vi "map_roi.vi"(8 "Error In":errorcluster, 9 "Image Properties":T2, 10 "Parameters":T1, 11 "ROI In":T3) -> (0 "Error Out":errorcluster, 3 "ROI Out":T3)   [LabVIEW 2019]
uses:
  image_property_cluster_typedef.ctl
  parameters_cluster_typedef.ctl
  xi_angles_enum_typedef.ctl
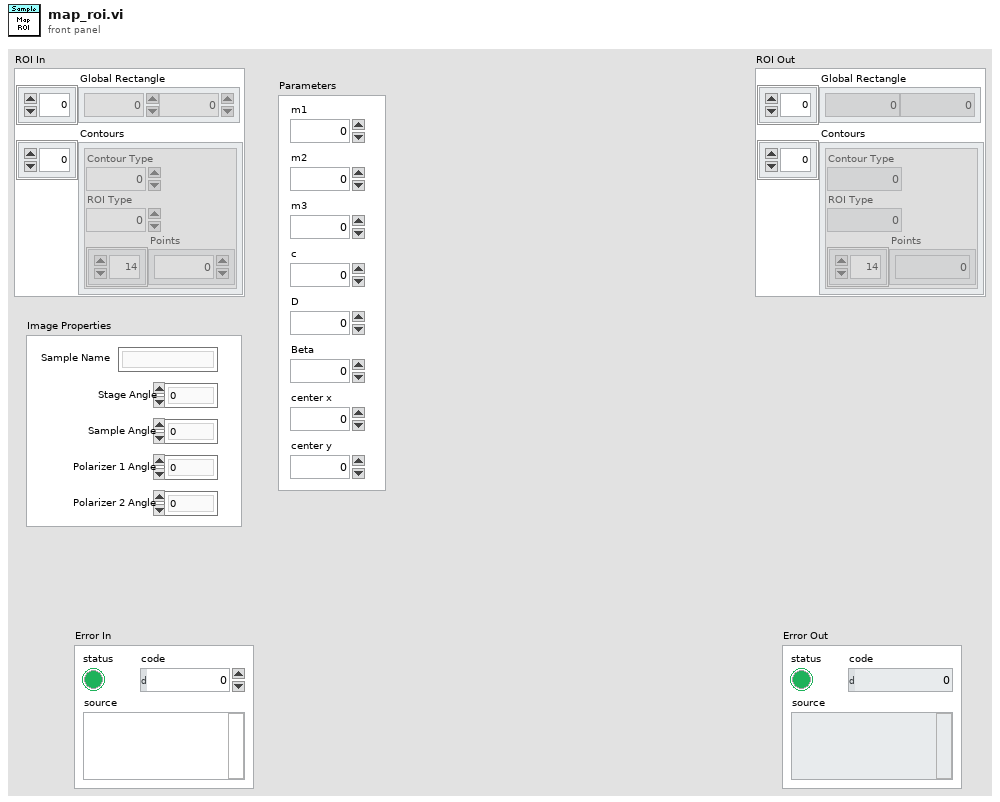
[diagram p1: front panel]
types:
  T1 = typedef "parameters_cluster_typedef.ctl" = cluster{"m1":dbl, "m2":dbl, "m3":dbl, "c":dbl, "D":dbl, "Beta":dbl, "center x":dbl, "center y":dbl}
  T2 = typedef "image_property_cluster_typedef.ctl" = cluster{"Stage Angle":dbl, "Sample Angle":dbl, "Polarizer 1 Angle":dbl, "Polarizer 2 Angle":dbl, "Sample Name":string}
  T3 = cluster{"Global Rectangle":i32[], "Contours":cluster{"Contour Type":u32, "ROI Type":u32, "Points":i32[]}[]}
  T4 = cluster{"Contour Type":u32, "ROI Type":u32, "Points":i32[]}
  T5 = typedef "xi_angles_enum_typedef.ctl" = enum16{"0", "45"}
  T6 = cluster{"Contour Type":u32, "ROI Type":u32, "Points":i32[]}[]
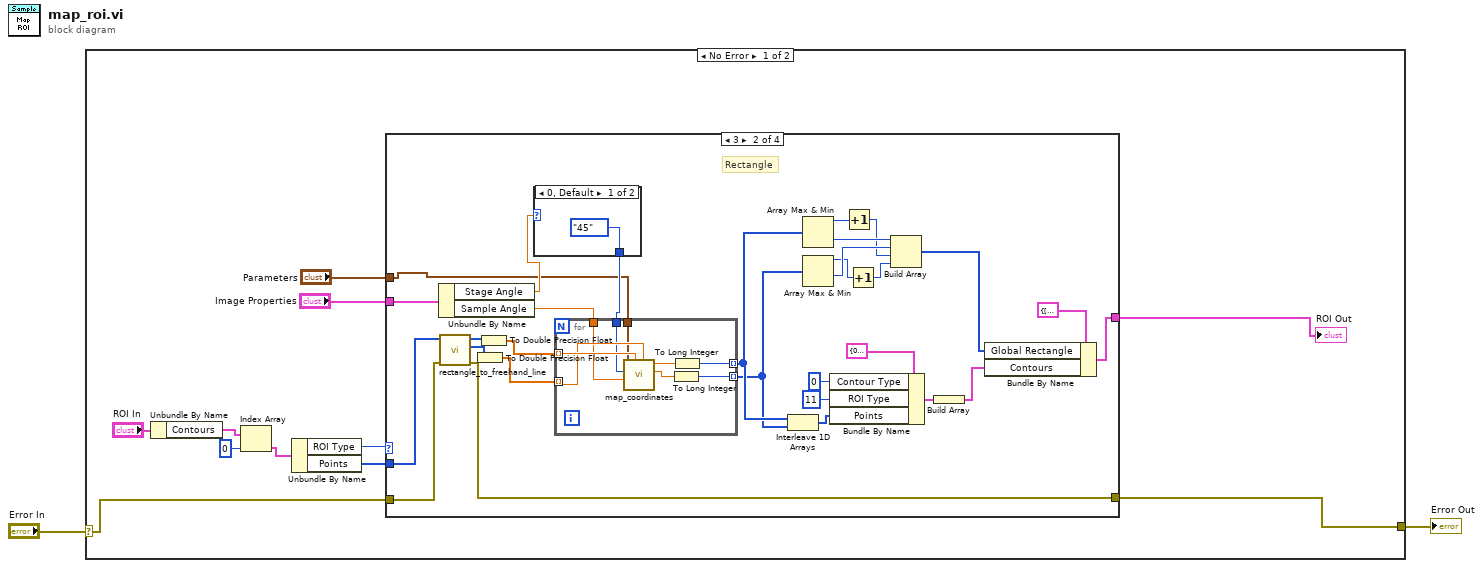
[diagram p0: block diagram]
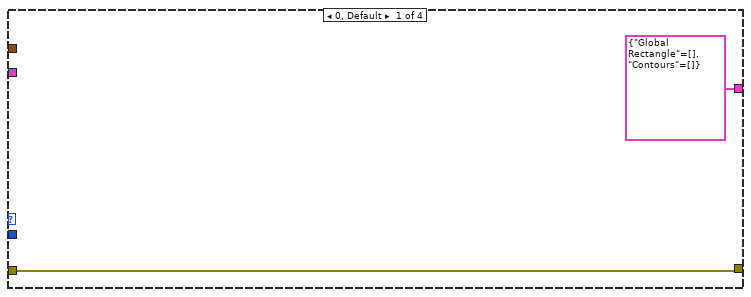
[diagram p2: hidden frame]
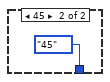
[diagram p3: hidden frame]
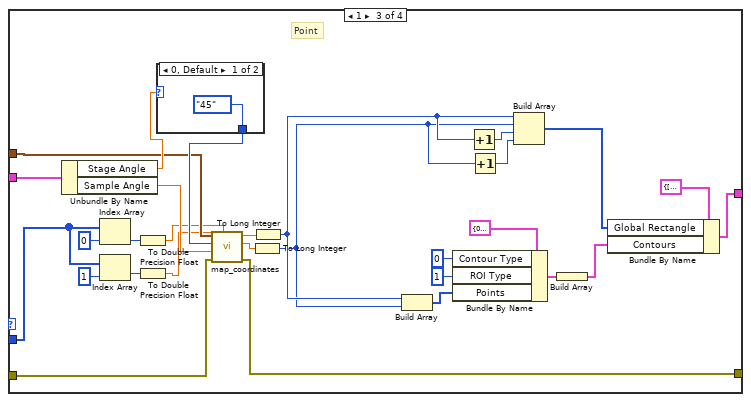
[diagram p4: hidden frame]
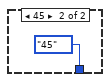
[diagram p5: hidden frame]
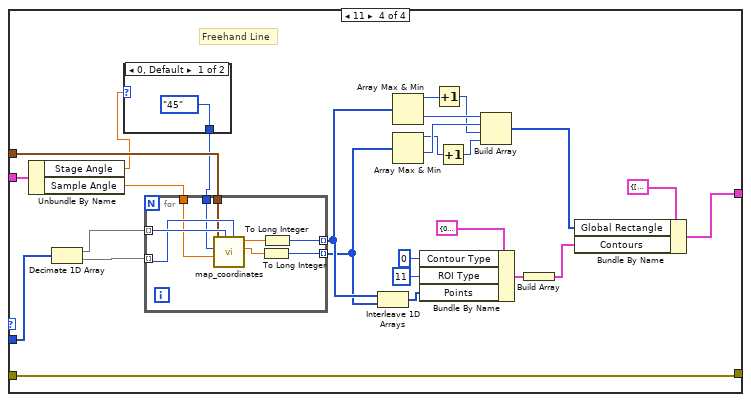
[diagram p6: hidden frame]
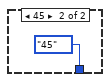
[diagram p7: hidden frame]
diagram:
  n1 = case shown="No Error" "Error In" {
    selector: "Error In" -> [w4 w124]
    tunnel: [w3 w124] -> w1
    frame No Error {
      n2 = Unbundle By Name("ROI In") -> ("Contours"=w12:T6)
      n3 = Index Array(array=w12, index=0) -> (element=w10:T4)
      n4 = Unbundle By Name(w10) -> ("ROI Type"=w9:u32, "Points"=w8:i32[])
      n5 = case shown="3" w9 {
        tunnel: w8 -> [_ w44 w72 w112]
        tunnel: "Parameters" -> [_ w23 w73 w107]
        tunnel: "Image Properties" -> [_ w22 w76 w109]
        tunnel: [T3 {"Global Rectangle"=[], "Contours"=[]} ("ROI Out") w17 w57 w105] -> w5
        tunnel: w4 -> [w14 w43 w65 w87]
        tunnel: [w14 w16 w56 w87] -> w3
        frame 0, Default {
        }
        frame 3 {
          # "Rectangle"
          n6 = Unbundle By Name(w22) -> ("Stage Angle"=w25:dbl, "Sample Angle"=w42:dbl)
          n7 = call "rectangle_to_freehand_line.vi"("Error In"=w43, "Input Rect"=w44) -> ("Error Out"=w16:errorcluster, "y"=w20:i32[], "x"=w21:i32[])  [unwired: 7 in]
          n8 = To Double Precision Float(number=w20) -> (double precision float=w18:dbl[])
          n9 = To Double Precision Float(number=w21) -> (double precision float=w19:dbl[])
          n10 = case shown="0, Default" w25 {
            tunnel: [xi_angles_enum_typedef."45" ("Xi From") xi_angles_enum_typedef."45" ("Xi From")] -> w24
            frame 0, Default {
            }
            frame 45 {
            }
          }
          n11 = for {
            tunnel: w19 -> [w55] mode=indexing
            tunnel: w18 -> [w54] mode=indexing
            tunnel: w42 -> [w53]
            tunnel: [w50] -> w34 mode=indexing
            tunnel: [w49] -> w33 mode=indexing
            tunnel: w23 -> [w48]
            tunnel: w24 -> [w47]
            n12 = call "map_coordinates.vi"("b"=w54, "a"=w55, "phi_in"=w53, "Xi From"=w47, "Parameters"=w48) -> ("b_pixel"=w51:dbl, "a_pixel"=w52:dbl)  [unwired: 4 in, 1 out]
            n13 = To Long Integer(number=w51) -> (32bit integer=w49:i32)
            n14 = To Long Integer(number=w52) -> (32bit integer=w50:i32)
          }
          n15 = Interleave 1D Arrays(w34, w33) -> (w37:i32[])
          n16 = Array Max & Min(array=w34) -> (max value=w30:i32, min value=w32:i32)  [unwired: 2 out]
          n17 = Array Max & Min(array=w33) -> (max value=w28:i32, min value=w31:i32)  [unwired: 2 out]
          n18 = Bundle By Name(cluster=T4 {"Contour Type"=0, "ROI Type"=0, "Points"=[]} ("Cluster"), "Contour Type"=u32 0, "ROI Type"=u32 11, "Points"=w37) -> (w36:T4)
          n19 = Increment(x=w30) -> (x+1=w29:i32)
          n20 = Increment(x=w28) -> (x+1=w27:i32)
          n21 = Build Array(w32, w31, w29, w27) -> (w26:i32[])
          n22 = Build Array(w36) -> (w35:T6)
          n23 = Bundle By Name(cluster=T3 {"Global Rectangle"=[387, 507, 423, 523], "Contours"=[{"Contour Type"=0, "ROI Type"=11, "Points"=[387, 521, 387, 520, 387, 519, 387, 518, 387, 517, 387, 516, 388, 516, 388, 515, 388, 514, 388, 513, 388, 512, 389, 512, 389, 511, 390, 511, 390, 510, 391, 510, 392, 510, 392, 509, 393, 509, 393, 508, 394, 508, 395, 508, 395, 507, 396, 507, 397, 507, 398, 508, 399, 508, 399, 509, 400, 509, 401, 509, 402, 509, 403, 509, 404, 509, 404, 510, 405, 510, 406, 510, 407, 510, 408, 510, 409, 510, 410, 510, 411, 510, 412, 510, 413, 510, 413, 511, 414, 511, 415, 511, 416, 511, 417, 512, 418, 512, 419, 512, 419, 513, 419, 514, 420, 514, 421, 514, 421, 515, 421, 516, 422, 517, 422, 518, 422, 519, 421, 519, 421, 520, 420, 520, 419, 520, 418, 520, 417, 520, 416, 520, 415, 520, 414, 520, 413, 520, 412, 520, 411, 520, 410, 520, 409, 520, 409, 521, 408, 521, 407, 521, 406, 521, 405, 521, 404, 521, 403, 521, 402, 521, 401, 521, 400, 521, 399, 521, 398, 521, 398, 522, 397, 522, 396, 522, 395, 522, 394, 522, 393, 522, 392, 522, 391, 522, 390, 522, 389, 522, 389, 522]}]} ("ROI Out"), "Global Rectangle"=w26, "Contours"=w35) -> (w17:T3)
        }
        frame 1 {
          # "Point"
          n24 = Unbundle By Name(w76) -> ("Stage Angle"=w77:dbl, "Sample Angle"=w75:dbl)
          n25 = Index Array(array=w72, index=0) -> (element=w69:i32)
          n26 = Index Array(array=w72, index=1) -> (element=w68:i32)
          n27 = To Double Precision Float(number=w69) -> (double precision float=w67:dbl)
          n28 = To Double Precision Float(number=w68) -> (double precision float=w66:dbl)
          n29 = case shown="0, Default" w77 {
            tunnel: [xi_angles_enum_typedef."45" ("Xi From") xi_angles_enum_typedef."45" ("Xi From")] -> w74
            frame 0, Default {
            }
            frame 45 {
            }
          }
          n30 = call "map_coordinates.vi"("b"=w66, "a"=w67, "Error In"=w65, "phi_in"=w75, "Xi From"=w74, "Parameters"=w73) -> ("Error Out"=w56:errorcluster, "b_pixel"=w63:dbl, "a_pixel"=w64:dbl)  [unwired: 3 in]
          n31 = To Long Integer(number=w63) -> (32bit integer=w58:i32)
          n32 = To Long Integer(number=w64) -> (32bit integer=w59:i32)
          n33 = Build Array(w59, w58) -> (w60:i32[])
          n34 = Bundle By Name(cluster=T4 {"Contour Type"=0, "ROI Type"=0, "Points"=[]} ("Cluster"), "Contour Type"=u32 0, "ROI Type"=u32 1, "Points"=w60) -> (w80:T4)
          n35 = Increment(x=w59) -> (x+1=w61:i32)
          n36 = Increment(x=w58) -> (x+1=w62:i32)
          n37 = Build Array(w59, w58, w61, w62) -> (w78:i32[])
          n38 = Build Array(w80) -> (w79:T6)
          n39 = Bundle By Name(cluster=T3 {"Global Rectangle"=[387, 507, 423, 523], "Contours"=[{"Contour Type"=0, "ROI Type"=11, "Points"=[387, 521, 387, 520, 387, 519, 387, 518, 387, 517, 387, 516, 388, 516, 388, 515, 388, 514, 388, 513, 388, 512, 389, 512, 389, 511, 390, 511, 390, 510, 391, 510, 392, 510, 392, 509, 393, 509, 393, 508, 394, 508, 395, 508, 395, 507, 396, 507, 397, 507, 398, 508, 399, 508, 399, 509, 400, 509, 401, 509, 402, 509, 403, 509, 404, 509, 404, 510, 405, 510, 406, 510, 407, 510, 408, 510, 409, 510, 410, 510, 411, 510, 412, 510, 413, 510, 413, 511, 414, 511, 415, 511, 416, 511, 417, 512, 418, 512, 419, 512, 419, 513, 419, 514, 420, 514, 421, 514, 421, 515, 421, 516, 422, 517, 422, 518, 422, 519, 421, 519, 421, 520, 420, 520, 419, 520, 418, 520, 417, 520, 416, 520, 415, 520, 414, 520, 413, 520, 412, 520, 411, 520, 410, 520, 409, 520, 409, 521, 408, 521, 407, 521, 406, 521, 405, 521, 404, 521, 403, 521, 402, 521, 401, 521, 400, 521, 399, 521, 398, 521, 398, 522, 397, 522, 396, 522, 395, 522, 394, 522, 393, 522, 392, 522, 391, 522, 390, 522, 389, 522, 389, 522]}]} ("ROI Out"), "Global Rectangle"=w78, "Contours"=w79) -> (w57:T3)
        }
        frame 11 {
          # "Freehand Line"
          n40 = Unbundle By Name(w109) -> ("Stage Angle"=w89:dbl, "Sample Angle"=w108:dbl)
          n41 = Decimate 1D Array(w112) -> (w111:i32[], w110:i32[])
          n42 = case shown="0, Default" w89 {
            tunnel: [xi_angles_enum_typedef."45" ("Xi From") xi_angles_enum_typedef."45" ("Xi From")] -> w88
            frame 0, Default {
            }
            frame 45 {
            }
          }
          n43 = for {
            tunnel: w111 -> [w123] mode=indexing
            tunnel: w110 -> [w122] mode=indexing
            tunnel: w108 -> [w121]
            tunnel: [w118] -> w98 mode=indexing
            tunnel: [w117] -> w97 mode=indexing
            tunnel: w107 -> [w116]
            tunnel: w88 -> [w115]
            n44 = call "map_coordinates.vi"("b"=w122, "a"=w123, "phi_in"=w121, "Xi From"=w115, "Parameters"=w116) -> ("b_pixel"=w119:dbl, "a_pixel"=w120:dbl)  [unwired: 4 in, 1 out]
            n45 = To Long Integer(number=w119) -> (32bit integer=w117:i32)
            n46 = To Long Integer(number=w120) -> (32bit integer=w118:i32)
          }
          n47 = Interleave 1D Arrays(w98, w97) -> (w101:i32[])
          n48 = Array Max & Min(array=w98) -> (max value=w94:i32, min value=w96:i32)  [unwired: 2 out]
          n49 = Array Max & Min(array=w97) -> (max value=w92:i32, min value=w95:i32)  [unwired: 2 out]
          n50 = Bundle By Name(cluster=T4 {"Contour Type"=0, "ROI Type"=0, "Points"=[]} ("Cluster"), "Contour Type"=u32 0, "ROI Type"=u32 11, "Points"=w101) -> (w100:T4)
          n51 = Increment(x=w94) -> (x+1=w93:i32)
          n52 = Increment(x=w92) -> (x+1=w91:i32)
          n53 = Build Array(w96, w95, w93, w91) -> (w90:i32[])
          n54 = Build Array(w100) -> (w99:T6)
          n55 = Bundle By Name(cluster=T3 {"Global Rectangle"=[387, 507, 423, 523], "Contours"=[{"Contour Type"=0, "ROI Type"=11, "Points"=[387, 521, 387, 520, 387, 519, 387, 518, 387, 517, 387, 516, 388, 516, 388, 515, 388, 514, 388, 513, 388, 512, 389, 512, 389, 511, 390, 511, 390, 510, 391, 510, 392, 510, 392, 509, 393, 509, 393, 508, 394, 508, 395, 508, 395, 507, 396, 507, 397, 507, 398, 508, 399, 508, 399, 509, 400, 509, 401, 509, 402, 509, 403, 509, 404, 509, 404, 510, 405, 510, 406, 510, 407, 510, 408, 510, 409, 510, 410, 510, 411, 510, 412, 510, 413, 510, 413, 511, 414, 511, 415, 511, 416, 511, 417, 512, 418, 512, 419, 512, 419, 513, 419, 514, 420, 514, 421, 514, 421, 515, 421, 516, 422, 517, 422, 518, 422, 519, 421, 519, 421, 520, 420, 520, 419, 520, 418, 520, 417, 520, 416, 520, 415, 520, 414, 520, 413, 520, 412, 520, 411, 520, 410, 520, 409, 520, 409, 521, 408, 521, 407, 521, 406, 521, 405, 521, 404, 521, 403, 521, 402, 521, 401, 521, 400, 521, 399, 521, 398, 521, 398, 522, 397, 522, 396, 522, 395, 522, 394, 522, 393, 522, 392, 522, 391, 522, 390, 522, 389, 522, 389, 522]}]} ("ROI Out"), "Global Rectangle"=w90, "Contours"=w99) -> (w105:T3)
        }
      }
      "ROI Out" <- w5
    }
    frame Error {
    }
  }
  "Error Out" <- w1
